vi "Test Process within Nested App Log Info Message.vi"(8 "error in (no error)":errorcluster, 11 "Test Case In":refnum<class "Logger Test.lvclass">) -> (0 "error out":errorcluster, 3 "Test Case Out":refnum<class "Logger Test.lvclass">)   [LabVIEW 2020, in "Logger Test.lvclass"]
uses:
  Logger Test.lvclass
  C:/Program Files (x86)/National Instruments/LabVIEW 2020/vi.lib/Asteme/LUnit/Test Case.lvclass
  Mock Log Handler/Mock Log Handler.lvclass
  C:/Users/anton/Documents/GitHub/Triarc-Framework/source/Framework/Logging/Logging.lvclass
  Mock Process/Mock Process.lvclass
  C:/Users/anton/Documents/GitHub/Triarc-Framework/source/Framework/Process/Process.lvclass
  Framework/Application/Application.lvclass
  Framework/Process/Process.lvclass/Process.ctl
  Framework/Application/Application.lvclass/Application.ctl
  <vilib>/Asteme/LUnit/Test Case.lvclass/Test Case.ctl
  <vilib>/Asteme/LUnit/LUnit Assertion Result.lvclass/LUnit Assertion Result.ctl
  Framework/Application/Private/Add Process to Map.vi
  Framework/Process/Protected/Messaging/Enqueue Message.vi
  Framework/Process/Protected/SubVIs/Set Context.vi
  Framework/Process/Public/Lifecycle/Get Lifecycle State.vi
  Framework/Process/Private/SubVIs/Wait for finish.vi
  Framework/Process/Private/SubVIs/Set Lifecycle State.vi
  <vilib>/Asteme/LUnit/Palette/Pass.vi
  <vilib>/Asteme/LUnit/Palette/Fail.vi
  <vilib>/Asteme/LUnit/Variant to string.vi
  <vilib>/Asteme/LUnit/Set Assertion Type.vi
  <vilib>/AdvancedString/1D String Array to Delimited String.vi
  Framework/Process/Community/Leave Process Loop.vi
  <vilib>/Asteme/LUnit/Add test result.vi
  <vilib>/Asteme/LUnit/LUnit Write Passed.vi
  <vilib>/Asteme/LUnit/LUnit Get Test Case.vi
  <vilib>/Asteme/LUnit/LUnit Write Message.vi
  <vilib>/Asteme/LUnit/LUnit Write Description.vi
  <vilib>/Asteme/LUnit/LUnit Write Assertion Type.vi
  <vilib>/Asteme/LUnit/Read Test Case Name.vi
  <vilib>/Utility/error.llb/Error Cluster From Error Code.vi
  Framework/Application/Private/Update Context for Owned Processes.vi
  <vilib>/Asteme/LUnit/Assertion Result/LUnit Get Test Name.vi
  <vilib>/Utility/Data Type/Get Type Information.vi
  <vilib>/Utility/LVClass/Get LV Class Name.vi
  <vilib>/Asteme/LUnit/LUnit Assertion Result.lvclass
  Framework/Process/Process.lvclass
  Framework/Logging/Logging.lvclass
  <vilib>/Asteme/LUnit/Test Case.lvclass
  Support/Framework Test Support.lvlib
  C:/Users/anton/Documents/GitHub/Triarc-Framework/source/Framework/Base/Base.lvclass
  C:/Users/anton/Documents/GitHub/Triarc-Framework/source/Framework/Error Handler Interface/Error Handler Interface.lvclass
  C:/Users/anton/Documents/GitHub/Triarc-Framework/source/Framework/Application/Application.lvclass
  C:/Users/anton/Documents/GitHub/Triarc-Framework/source/Framework Test/Logger Test/Logger Test.lvclass
  C:/Users/anton/Documents/GitHub/Triarc-Framework/source/Framework Test/Mock Process/Mock Process.lvclass
  C:/Users/anton/Documents/GitHub/Triarc-Framework/source/Framework/Helper Loop/Helper Loop.lvclass
  C:/Users/anton/Documents/GitHub/Triarc-Framework/source/Framework Test/Mock Log Handler/Mock Log Handler.lvclass
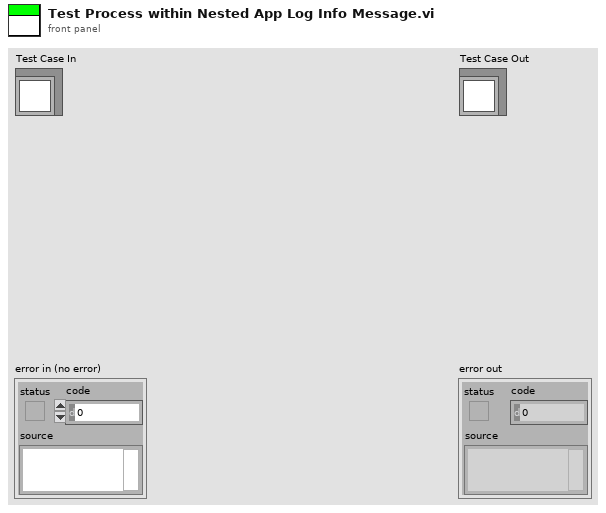
[diagram p1: front panel]
types:
  T1 = typedef "Mock Log Handler.lvclass/Log Entry.ctl" = cluster{"Level":string, "Source":string, "Message":string}
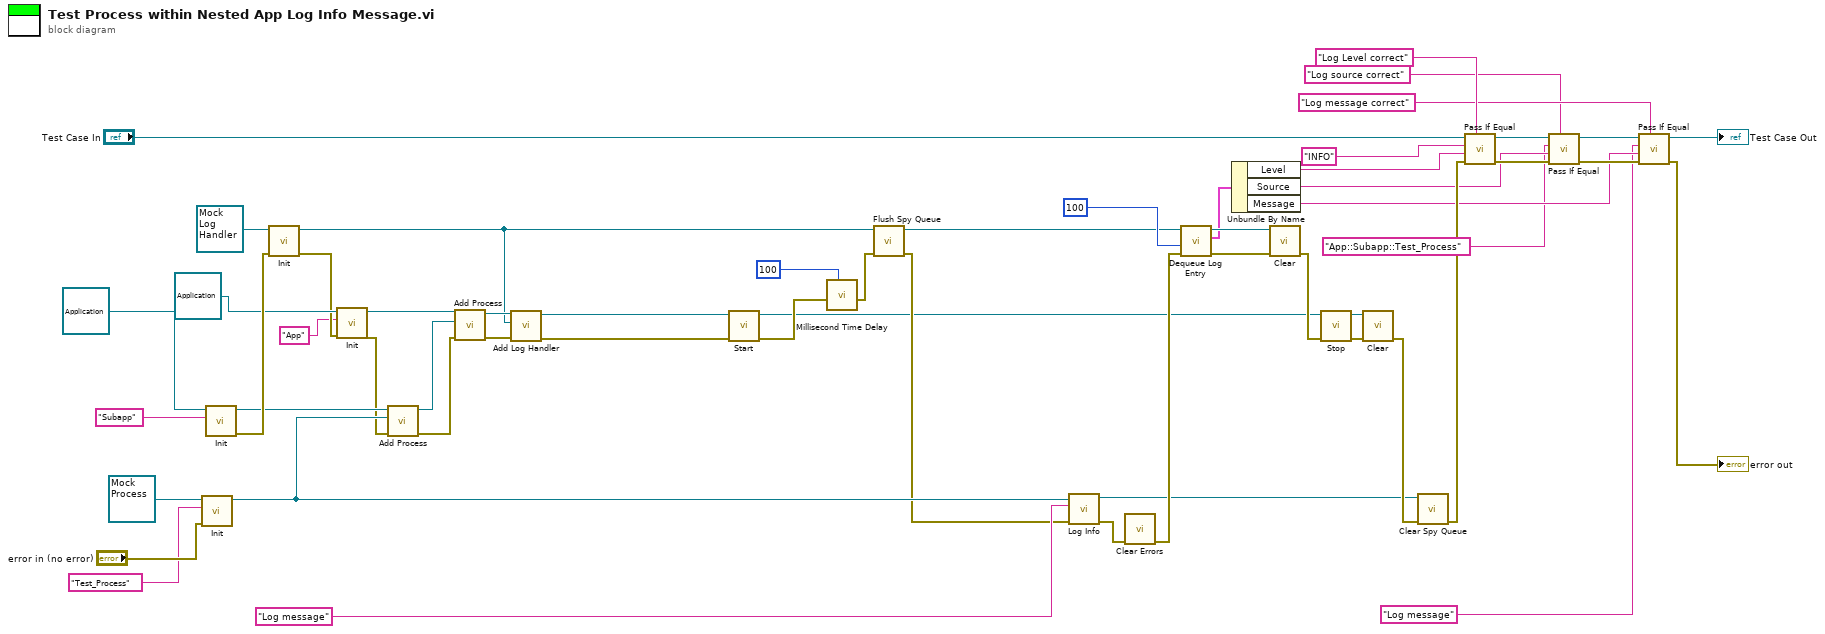
[diagram p0: block diagram]
diagram:
  n1 = call-dynamic "Init.vi"("error in (no error)"="error in (no error)", "Name"="Test_Process", "Mock Process In"=refnum<class "Mock Process.lvclass"> refnum) -> ("Mock Process Out"=w17:refnum<class "Mock Process.lvclass">)  [unwired: 7 in, 1 out]
  n2 = call-dynamic "Init.vi"("Name"="Subapp", "Process In"=refnum<class "Application.lvclass"> refnum ("Application.lvclass")) -> ("error out"=w51:errorcluster, "Process Out"=w9:refnum<class "Application.lvclass">)  [unwired: 8 in]
  n3 = call-dynamic "Init.vi"("error in (no error)"=w51, "Mock Log Handler In"=refnum<class "Mock Log Handler.lvclass"> refnum ("Mock Log Handler.lvclass")) -> ("error out"=w14:errorcluster, "Mock Log Handler Out"=w10:refnum<class "Mock Log Handler.lvclass">)  [unwired: 8 in]
  n4 = call-dynamic "Init.vi"("error in (no error)"=w14, "Name"="App", "Process In"=refnum<class "Application.lvclass"> refnum ("Application.lvclass")) -> ("error out"=w7:errorcluster, "Process Out"=w13:refnum<class "Application.lvclass">)  [unwired: 7 in]
  n5 = call "Add Process.vi"("error in (no error)"=w7, "Process"=w17, "Rig In"=w9) -> ("error out"=w6:errorcluster, "Rig Out"=w8:refnum<class "Application.lvclass">)  [unwired: 7 in]
  n6 = call "Add Process.vi"("error in (no error)"=w6, "Process"=w8, "Rig In"=w13) -> ("error out"=w11:errorcluster, "Rig Out"=w12:refnum<class "Application.lvclass">)  [unwired: 7 in]
  n7 = call "Add Log Handler.vi"("error in (no error)"=w11, "Log Handler"=w10, "Process In"=w12) -> ("error out"=w5:errorcluster, "Process Out"=w3:refnum<class "Application.lvclass">)  [unwired: 7 in]
  n8 = call "Start.vi"("error in (no error)"=w5, "Process In"=w3) -> ("error out"=w4:errorcluster, "Process Out"=w2:refnum<class "Application.lvclass">)  [unwired: 8 in]
  n9 = call "Millisecond Time Delay.vi"("milliseconds to wait"=u32 100, "error in (no error)"=w4) -> ("error out"=w19:errorcluster)  [unwired: 7 in]
  n10 = call "Flush Spy Queue.vi"("error in (no error)"=w19, "Mock Log Handler in"=w10) -> ("error out"=w16:errorcluster, "Mock Log Handler out"=w20:refnum<class "Mock Log Handler.lvclass">)  [unwired: 7 in, 1 out]
  n11 = call "Log Info.vi"("error in (no error)"=w16, "Message"="Log message", "Logging In"=w17) -> ("error out"=w32:errorcluster, "Logging Out"=w22:refnum<class "Mock Process.lvclass">)  [unwired: 7 in]
  n12 = call <vilib>:"Clear Errors.vi"("error in (no error)"=w32) -> ("error out"=w31:errorcluster)  [unwired: 5 in, 1 out]
  n13 = call "Dequeue Log Entry.vi"("error in (no error)"=w31, "timeout in ms (-1)"=100, "Mock Log Handler in"=w20) -> ("error out"=w49:errorcluster, "Entry"=w46:T1, "Mock Log Handler out"=w50:refnum<class "Mock Log Handler.lvclass">)  [unwired: 5 in, 1 out]
  n14 = Unbundle By Name(w46) -> ("Level"=w45:string, "Source"=w35:string, "Message"=w34:string)
  n15 = call-dynamic "Clear.vi"("error in (no error)"=w49, "Mock Log Handler In"=w50) -> ("error out"=w47:errorcluster)  [unwired: 8 in, 1 out]
  n16 = call "Stop.vi"("error in (no error)"=w47, "Process In"=w2) -> ("error out"=w24:errorcluster, "Process Out"=w23:refnum<class "Application.lvclass">)  [unwired: 7 in, 1 out]
  n17 = call-dynamic "Clear.vi"("error in (no error)"=w24, "Application In"=w23) -> ("error out"=w53:errorcluster)  [unwired: 8 in, 1 out]
  n18 = call-dynamic "Clear Spy Queue.vi"("error in (no error)"=w53, "Mock Process In"=w22) -> ("error out"=w39:errorcluster)  [unwired: 8 in, 1 out]
  n19 = call <vilib>:"Pass If Equal.vi"("Description"="Log Level correct", "error in (no error)"=w39, "Actual"=w45, "Expected"="INFO", "Test Case In"="Test Case In") -> ("error out"=w41:errorcluster, "Test Case Out"=w55:refnum<class "Logger Test.lvclass">)  [unwired: 5 in]
  n20 = call <vilib>:"Pass If Equal.vi"("Description"="Log source correct", "error in (no error)"=w41, "Actual"=w35, "Expected"="App::Subapp::Test_Process" ("Name"), "Test Case In"=w55) -> ("error out"=w40:errorcluster, "Test Case Out"=w43:refnum<class "Logger Test.lvclass">)  [unwired: 5 in]
  n21 = call <vilib>:"Pass If Equal.vi"("Description"="Log message correct", "error in (no error)"=w40, "Actual"=w34, "Expected"="Log message" ("Message"), "Test Case In"=w43) -> ("error out"=→"error out":errorcluster, "Test Case Out"=→"Test Case Out":refnum<class "Logger Test.lvclass">)  [unwired: 5 in]
